vi "SnoDetectMotion.vi"(11 "Motor Values":dbl[](array[numeric])) -> (3 "Boolean":bool)   [LabVIEW 2013]
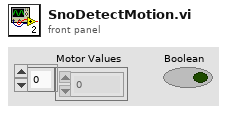
[diagram p1: front panel]
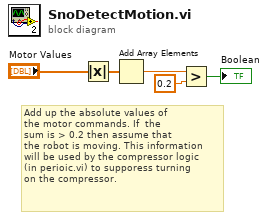
[diagram p0: block diagram]
diagram:
  # "Add up the absolute values of\nthe motor commands. If  the\nsum is > 0.2 then assume that\nthe robot is moving. This information\nwill be used by the compressor logic\n(in perioic.vi) to supporess turning\non the compressor."
  n1 = Absolute Value(x="Motor Values") -> (abs(x)=w2:dbl[])
  n2 = Add Array Elements(numeric array=w2) -> (sum=w4:dbl)
  n3 = Greater?(x=w4, y=0.2) -> (0:→"Boolean":bool)
